vi "example test.vi"() -> ()   [LabVIEW 2013, in "EthernetIP tests.lvlib"]
uses:
  EthernetIP tests.lvlib
  configuration/EthernetIP configuration.lvclass
  execution/EthernetIP runtime.lvclass
  configuration/assembly type.ctl
  <vilib>/NI/Tag Bus/tag/Data Type.ctl
  <vilib>/NI/Tag Bus/dictionary/data dictionary.lvclass/data dictionary.ctl
  <vilib>/NI/Tag Bus/dictionary/lookup polymorphs/locate U16.vi
  <vilib>/NI/Tag Bus/table/data polymorphs/write one/write U16.vi
  <vilib>/NI/Tag Bus/table/data polymorphs/read one/read U16.vi
  <vilib>/NI/Tag Bus/dictionary/search/find data index.vi
  <vilib>/NI/Tag Bus/dictionary/search/search string list.vi
  <vilib>/NI/Tag Bus/dictionary/tag not found.vi
  <vilib>/NI/Tag Bus/tag/tag descriptor.lvclass
  <vilib>/NI/Tag Bus/dictionary/data dictionary.lvclass
  <vilib>/NI/Tag Bus/table/data table.lvlib
  channel/EthernetIP Channel.lvclass
  <vilib>/NI/Configuration Framework/serializable configuration/NISE_CEF_serializable configuration.lvclass
panel:
  in  "big endian?":bool=TRUE
  in  "stop":bool
  in  "value TX":u16(slide)=42 scale=0.0..16000.0
  out "value RX":u16(slide) scale=0.0..16000.0
  out "final error":errorcluster
  out "output error":errorcluster
  out "input error":errorcluster
  out "output lookup error":errorcluster
  out "no data written":bool
  out "input lookup error":errorcluster
  out "init error":errorcluster
  out "correct execution settings":bool
  out "serialization problem":errorcluster
  out "invalid configuration":errorcluster
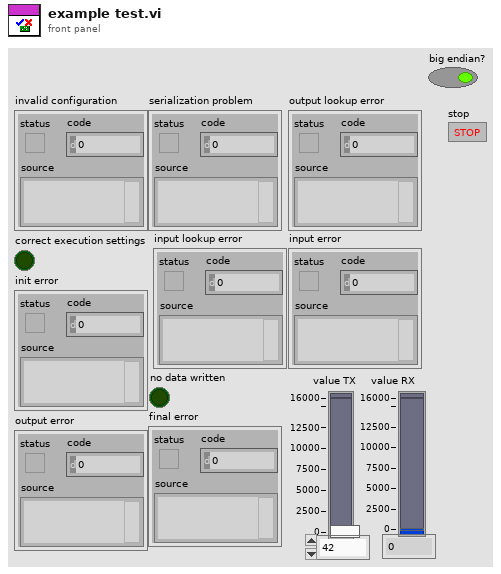
[diagram p1: front panel]
types:
  T1 = typedef "tag bus.lvlib/tag descriptor.lvclass/Data Type.ctl" = enum16{"Double", "Single", "I64", "I32", "I16", "I8", "U64", "U32", "U16", "U8", "Boolean", "String", "Array of Double", "Array of Single", "Array of I64", "Array of I32", "Array of I16", "Array of I8", "Array of U64", "Array of U32", "Array of U16", "Array of U8", "Array of Boolean", "Array of String"}
  T2 = typedef "EthernetIP configuration.lvclass/assembly type.ctl" = enum32{"Producing", "Consuming"}
  T3 = typedef "TBM channel.lvclass/data tables.ctl" = cluster{"input data":T4, "processing parameter":T4, "processing result":T4, "output data":T4}
  T4 = typedef "tag bus.lvlib/dictionary table pair.ctl" = cluster{"data dictionary":refnum<class "data dictionary.lvclass">, "data table":T5}
  T5 = typedef "tag bus.lvlib/data table.lvlib/data table.ctl" = cluster{"Double":dbl[], "Single":sgl[], "I64":i64[], "I32":i32[], "I16":i16[], "I8":i8[], "U64":u64[], "U32":u32[], "U16":u16[], "U8":u8[], "Boolean":bool[], "String":string[], "Array of Double":cluster{"DBL Array":dbl[]}[], "Array of Single":cluster{"SGL Array":sgl[]}[], "Array of I64":cluster{"I64 Array":i64[]}[], "Array of I32":cluster{"I32 Array":i32[]}[], "Array of I16":cluster{"I16 Array":i16[]}[], "Array of I8":cluster{"I8 Array":i8[]}[], "Array of U64":cluster{"U64 Array":u64[]}[], "Array of U32":cluster{"U32 Array":u32[]}[], "Array of U16":cluster{"U16 Array":u16[]}[], "Array of U8":cluster{"U8 Array":u8[]}[], "Array of Boolean":cluster{"Boolean Array":bool[]}[], "Array of String":cluster{"String Array":string[]}[]}
  T6 = typedef "TBM module execution interface.lvclass/execution settings.ctl" = cluster{"reads inputs":bool, "processes data":bool, "writes outputs":bool}
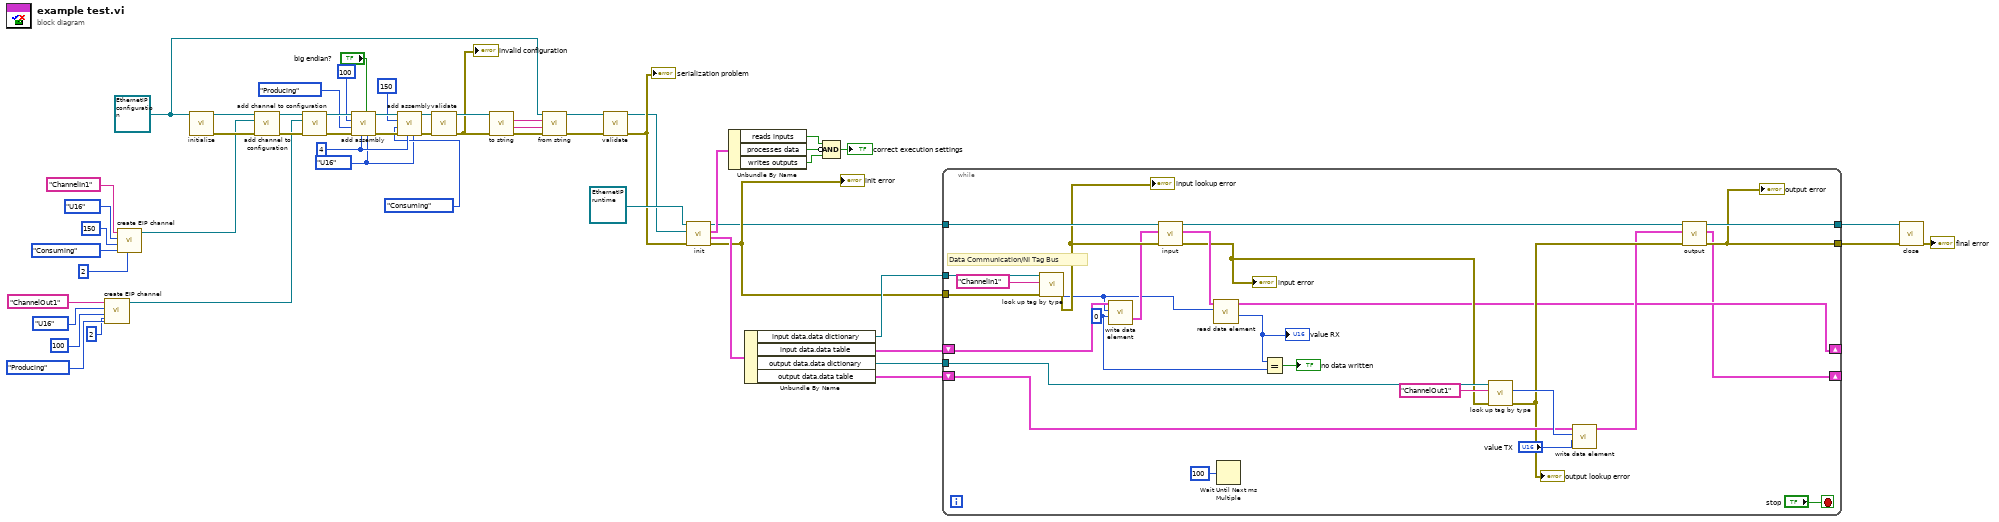
[diagram p0: block diagram]
diagram:
  w2 = Data_Type."U16" ("data type")
  w8 = u32 4 ("Size (bytes)")
  w1 = refnum<class "EthernetIP configuration.lvclass"> refnum ("tag bus configurable plugin module configuration")
  n1 = call "create EIP channel.vi"("element"=2 ("byte index"), "Type"=assembly_type."Producing", "Instance ID"=u32 100, "data type"=Data_Type."U16", "name"="ChannelOut1" ("channel name")) -> ("EthernetIP Channel out"=w19:refnum<class "EthernetIP Channel.lvclass">)  [unwired: 6 in]
  n2 = call "create EIP channel.vi"("element"=2 ("byte index"), "Type"=assembly_type."Consuming", "Instance ID"=u32 150, "data type"=Data_Type."U16", "name"="ChannelIn1" ("channel name")) -> ("EthernetIP Channel out"=w13:refnum<class "EthernetIP Channel.lvclass">)  [unwired: 6 in]
  n3 = call <vilib>:"initialize.vi"("configuration in"=w1) -> ("error out"=w27:errorcluster, "configuration out"=w28:refnum<class "EthernetIP configuration.lvclass">)  [unwired: 8 in, 1 out]
  n4 = call "add channel to configuration.vi"("error in"=w27, "TBM channel in"=w13, "EthernetIP configuration in"=w28) -> ("error out"=w29:errorcluster, "EthernetIP configuration out"=w30:refnum<class "EthernetIP configuration.lvclass">)  [unwired: 7 in]
  n5 = call "add channel to configuration.vi"("error in"=w29, "TBM channel in"=w19, "EthernetIP configuration in"=w30) -> ("error out"=w26:errorcluster, "EthernetIP configuration out"=w11:refnum<class "EthernetIP configuration.lvclass">)  [unwired: 7 in]
  n6 = call "add assembly.vi"("data type"=w2, "big endian?"="big endian?", "size (elements)"=w8, "error in"=w26, "Type"=assembly_type."Producing", "instance ID"=u32 100 ("Instance ID"), "EthernetIP configuration in"=w11) -> ("error out"=w12:errorcluster, "EthernetIP configuration out"=w9:refnum<class "EthernetIP configuration.lvclass">)  [unwired: 3 in]
  n7 = call "add assembly.vi"("data type"=w2, "size (elements)"=w8, "error in"=w12, "Type"=assembly_type."Consuming", "instance ID"=u32 150 ("Instance ID"), "EthernetIP configuration in"=w9) -> ("error out"=w10:errorcluster, "EthernetIP configuration out"=w25:refnum<class "EthernetIP configuration.lvclass">)  [unwired: 4 in]
  n8 = call-dynamic "validate.vi"("error in"=w10, "EthernetIP configuration in"=w25) -> ("error out"=w54:errorcluster, "EthernetIP configuration out"=w55:refnum<class "EthernetIP configuration.lvclass">)  [unwired: 8 in]
  "invalid configuration" <- w54
  n9 = call-dynamic "to string.vi"("error in"=w54, "EthernetIP configuration in"=w55) -> ("error out"=w51:errorcluster, "data"=w52:string, "version"=w53:string)  [unwired: 6 in, 1 out]
  n10 = call-dynamic "from string.vi"("error in"=w51, "data"=w52, "version"=w53, "EthernetIP configuration in"=w1) -> ("error out"=w49:errorcluster, "EthernetIP configuration out"=w50:refnum<class "EthernetIP configuration.lvclass">)  [unwired: 6 in]
  n11 = call-dynamic "validate.vi"("error in"=w49, "EthernetIP configuration in"=w50) -> ("error out"=w47:errorcluster, "EthernetIP configuration out"=w46:refnum<class "EthernetIP configuration.lvclass">)  [unwired: 8 in]
  "serialization problem" <- w47
  n12 = call-dynamic "init.vi"("error in"=w47, "TBM module configuration in"=w46, "EthernetIP runtime in"=refnum<class "EthernetIP runtime.lvclass"> refnum ("tag bus configurable plugin module")) -> ("error out"=w38:errorcluster, "data allocations"=w40:T3, "execution settings"=w45:T6, "EthernetIP runtime out"=w36:refnum<class "EthernetIP runtime.lvclass">)  [unwired: 5 in]
  "init error" <- w38
  n13 = Unbundle By Name(w45) -> ("reads inputs"=w42:bool, "processes data"=w44:bool, "writes outputs"=w43:bool)
  n14 = Unbundle By Name(w40) -> ("input data.data dictionary"=w39:refnum<class "data dictionary.lvclass">, "input data.data table"=w37:T5, "output data.data dictionary"=w35:refnum<class "data dictionary.lvclass">, "output data.data table"=w34:T5)
  n15 = Compound Arithmetic op=AND(w42, invert w44, w43) -> (→"correct execution settings":bool)
  n16 = while {
    tunnel: w39 -> [w82]
    tunnel: w38 -> [w81]
    tunnel: w36 -> [w78]
    tunnel: w35 -> [w71]
    tunnel: [w62] -> w33
    tunnel: [w61] -> w32
    shift-right: [w58] -> _
    shift-left: w34 -> [w68]
    shift-right: [w59] -> _
    shift-left: w37 -> [w79]
    stop <- "stop" stop-if-true
    w60 = u16 0 ("value")
    # "Data Communication/NI Tag Bus"
    n17 = call-poly <vilib>:"look up tag by type.vi"("error in"=w81, "name"="ChannelIn1" ("channel name"), "data dictionary in"=w82) -> ("error out"=w77:errorcluster, "index"=w74:i32)  [unwired: 6 in, 1 out]
    "input lookup error" <- w77
    n18 = call-poly <vilib>:"write data element.vi"("value"=w60, "index"=w74, "data table in"=w79) -> ("data table out"=w76:T5)  [unwired: 8 in]
    n19 = call-dynamic "input.vi"("error in"=w77, "data table in"=w76, "EthernetIP runtime in"=w78) -> ("error out"=w67:errorcluster, "data table out"=w75:T5, "EthernetIP runtime out"=w64:refnum<class "EthernetIP runtime.lvclass">)  [unwired: 6 in]
    "input error" <- w67
    n20 = call-poly <vilib>:"read data element.vi"("index"=w74, "data table in"=w75) -> ("value"=w73:u16, "data table out"=w59:T5)  [unwired: 8 in]
    "value RX" <- w73
    n21 = Wait Until Next ms Multiple(millisecond multiple=u32 100) -> ()  [unwired: 1 out]
    n22 = Equal?(x=w73, y=w60) -> (x = y?=→"no data written":bool)
    n23 = call-poly <vilib>:"look up tag by type.vi"("error in"=w67, "name"="ChannelOut1" ("channel name"), "data dictionary in"=w71) -> ("error out"=w65:errorcluster, "index"=w69:i32)  [unwired: 6 in, 1 out]
    "output lookup error" <- w65
    n24 = call-poly <vilib>:"write data element.vi"("value"="value TX", "index"=w69, "data table in"=w68) -> ("data table out"=w63:T5)  [unwired: 8 in]
    n25 = call-dynamic "output.vi"("error in"=w65, "data table in"=w63, "EthernetIP runtime in"=w64) -> ("error out"=w61:errorcluster, "data table out"=w58:T5, "EthernetIP runtime out"=w62:refnum<class "EthernetIP runtime.lvclass">)  [unwired: 6 in]
    "output error" <- w61
  }
  n26 = call-dynamic "close.vi"("error in"=w32, "EthernetIP runtime in"=w33) -> ("error out"=→"final error":errorcluster)  [unwired: 9 in]
